vi "Wait for Start.vi"(8 "error in (no error)":errorcluster, 11 "Actor API in":refnum<class "Actor API.lvclass">) -> (0 "error out":errorcluster, 3 "Actor API out":refnum<class "Actor API.lvclass">)   [LabVIEW 2020, in "Artifex.lvlib" / "Actor API.lvclass"]
uses:
  Actor API.lvclass
  Actor API.lvclass/Actor API.ctl
  Stop Msg/Stop Msg.lvclass
  Priority Message Queue/Priority Message Queue.lvclass
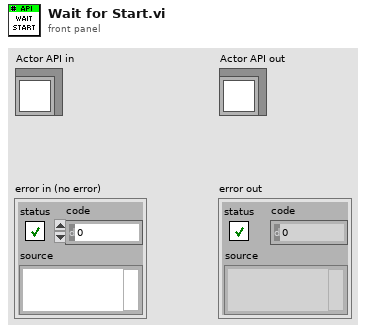
[diagram p1: front panel]
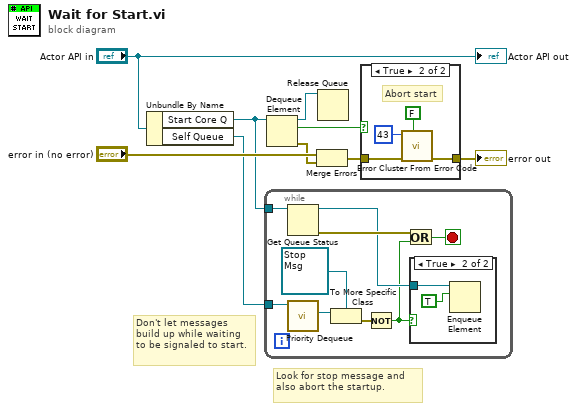
[diagram p0: block diagram]
diagram:
  # "Look for stop message and also abort the startup."
  # "Don't let messages build up while waiting to be signaled to start."
  n1 = Unbundle By Name("Actor API in") -> ("Start Core Q"=w3:refnum<queue>, "Self Queue"=w2:refnum<class "Priority Message Queue.lvclass">)
  n2 = while {
    tunnel: w3 -> [w18]
    tunnel: w2 -> [w16]
    stop <- w11 stop-if-true
    n3 = Get Queue Status(queue=w18) -> (queue out=w12:refnum<queue>, error out=w17:errorcluster)  [unwired: 2 in, 6 out]
    n4 = call "Priority Dequeue.vi"("Priority Message Queue in"=w16) -> ("Message"=w15:refnum<class "Message.lvclass">)  [unwired: 6 in, 4 out]
    n5 = To More Specific Class(target class=refnum<class "Stop Msg.lvclass"> refnum ("Artifex.lvlib:Stop Msg.lvclass"), reference=w15) -> (error out=w13:errorcluster)  [unwired: 1 in, 1 out]
    n6 = Not(x=w13) -> (.not. x?=w10:bool)
    n7 = Or(x=w17, y=w10) -> (x .or. y?=w11:bool)
    n8 = case shown="True" w10 {
      tunnel: w12 -> [_ w20]
      frame False {
      }
      frame True {
        n9 = Enqueue Element(queue=w20, element=TRUE) -> ()  [unwired: 2 in, 3 out]
      }
    }
  }
  n10 = Dequeue Element(queue=w3) -> (queue out=w1:refnum<queue>, element=w8:bool, error out=w5:errorcluster)  [unwired: 2 in, 1 out]
  n11 = Merge Errors("error in (no error)", w5) -> (w6:errorcluster)
  n12 = Release Queue(queue=w1) -> ()  [unwired: 2 in, 3 out]
  n13 = case shown="True" w8 {
    tunnel: w6 -> [w21 w25]
    tunnel: [w21 w22] -> w7
    frame False {
    }
    frame True {
      # "Abort start"
      n14 = call <vilib>:"Error Cluster From Error Code.vi"("show call chain? (False)"=FALSE, "error in (no error)"=w25, "error code (0)"=43) -> ("error out"=w22:errorcluster)  [unwired: 6 in]
    }
  }
  "error out" <- w7
  "Actor API out" <- "Actor API in"
